vi "Write Prompt to add new approved file to project_(T).vi"(8 "error in":errorcluster, 10 "Prompt New Approved File":bool, 11 "Options in":refnum<class "Options.lvclass">) -> (0 "error out":errorcluster, 3 "Options out":refnum<class "Options.lvclass">)   [LabVIEW 2020, in "Approval Tests.lvlib" / "Options.lvclass"]
uses:
  Options.lvclass
  Options.lvclass/Options.ctl
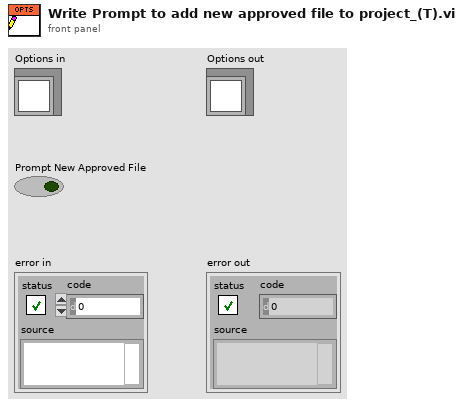
[diagram p1: front panel]
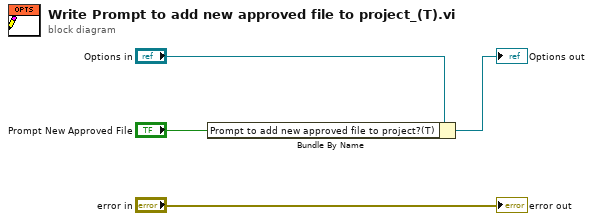
[diagram p0: block diagram]
diagram:
  n1 = Bundle By Name(cluster="Options in", "Prompt to add new approved file to project?(T)"="Prompt New Approved File") -> (→"Options out":refnum<class "Options.lvclass">)
  "error out" <- "error in"
